vi "Write txt.vi"(7 "Enum":T1, 8 "error in":errorcluster, 9 "Zone":i32, 10 "Status":string, 11 "file path":path) -> (0 "error out":errorcluster)   [LabVIEW 2013]
doc: "This subVI is initialize the file path, writing the data to the security log.txt and release the file path."
uses:
  Controls/Write txt.ctl
  <vilib>/Utility/file.llb/Write To Spreadsheet File (string).vi
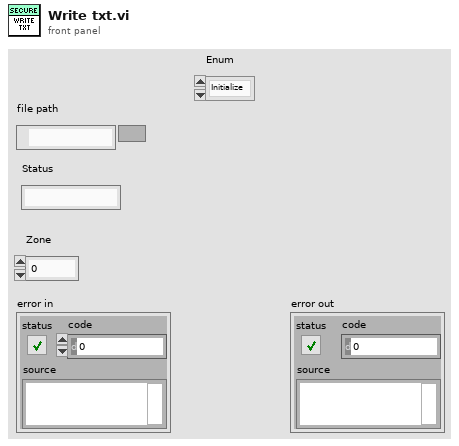
[diagram p1: front panel]
types:
  T1 = typedef "Write txt.ctl" = enum16{"Initialize", "Write", "Stop"}
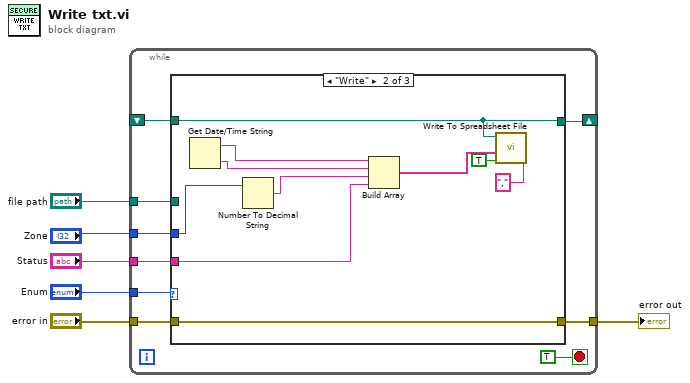
[diagram p0: block diagram]
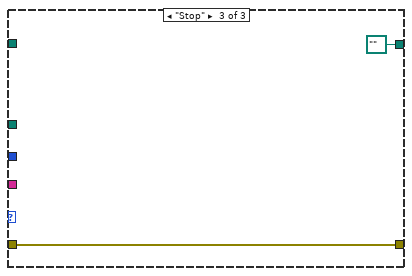
[diagram p3: hidden frame]
diagram:
  n1 = while {
    tunnel: "Enum" -> [w15]
    tunnel: "file path" -> [w13]
    shift-right: [w14] -> _
    shift-left: _ -> [w12]
    tunnel: "Status" -> [w11]
    tunnel: "error in" -> [w9]
    tunnel: [w8] -> w6
    tunnel: "Zone" -> [w7]
    stop <- TRUE stop-if-true
    n2 = case shown="\"Write\"" w15 {
      tunnel: [w17 w22 path "" ("file path")] -> w14
      tunnel: w13 -> [w17 _ _]
      tunnel: w12 -> [_ w22 _]
      tunnel: w11 -> [_ w25 _]
      tunnel: w9 -> [w16 w21 w28]
      tunnel: [w16 w21 w28] -> w8
      tunnel: w7 -> [_ w18 _]
      frame "Initialize", Default {
      }
      frame "Write" {
        n3 = Get Date/Time String() -> (date string=w27:string, time string=w26:string)  [unwired: 3 in]
        n4 = Number To Decimal String(number=w18) -> (decimal integer string=w20:string)  [unwired: 1 in]
        n5 = Build Array(w27, w26, w20, w25) -> (w24:string[])
        n6 = call-poly <vilib>:"Write To Spreadsheet File.vi"("delimiter (\\t)"="," ("delimiter (\\t)"), "append to file? (new file:F)"=TRUE, "1D data"=w24, "file path (dialog if empty)"=w22) -> ()  [unwired: 4 in, 1 out]
      }
      frame "Stop" {
      }
    }
  }
  "error out" <- w6
